vi "Keithley 6221-2182.vi"() -> ()   [LabVIEW 2018]
doc: "Stores specified measurements in buffer and reads the contents of the buffer as well as its statistics."
uses:
  <instrlib>/Keithley 622x LV 2009/Configure/Source/Typedefs/KE622x -- Current Range.ctl
  <instrlib>/Keithley 622x LV 2009/Configure/Source/Typedefs/KE622x -- Current Ranges.ctl
  <instrlib>/Keithley 622x LV 2009/Configure/Source/Typedefs/KE622x -- Lin Log Sweep Params.ctl
  <instrlib>/Keithley 622x LV 2009/Configure/Source/Typedefs/KE622x -- Source Delay.ctl
  <instrlib>/Keithley 622x LV 2009/Configure/Source/Typedefs/KE622x -- Current Level.ctl
  <instrlib>/Keithley 622x LV 2009/Typedefs/KE622x -- On Off Control.ctl
  <instrlib>/Keithley 622x LV 2009/Configure/Source/Typedefs/KE622x -- Voltage Limit.ctl
  <instrlib>/Keithley 622x LV 2009/Configure/Output/Typedefs/KE6221 -- Output Response.ctl
  <instrlib>/Keithley 622x LV 2009/Configure/Source/Typedefs/KE622x -- Sweep Type.ctl
  <instrlib>/Keithley 622x LV 2009/Configure/Trigger/Typedefs/KE6221 -- Arm Trig Wave Trig Params.ctl
  <instrlib>/Keithley 622x LV 2009/Configure/Trigger/Low Level/Typedefs/KE622x -- Arm Source.ctl
  <instrlib>/Keithley 622x LV 2009/Configure/Trigger/Low Level/Typedefs/KE622x -- Trig Link Line.ctl
  <instrlib>/Keithley 622x LV 2009/Configure/Trigger/Low Level/Typedefs/KE622x -- Arm Timer Interval.ctl
  <instrlib>/Keithley 622x LV 2009/Configure/Trigger/Low Level/Typedefs/KE622x -- Arm Output Mode.ctl
  <instrlib>/Keithley 622x LV 2009/Configure/Trigger/Low Level/Typedefs/KE622x -- Trig Source.ctl
  <instrlib>/Keithley 622x LV 2009/Configure/Trigger/Low Level/Typedefs/KE622x -- Trig Output Mode.ctl
  <instrlib>/Keithley 622x LV 2009/Configure/6221 Wave/Low Level/Typedefs/KE6221 -- Wave Extern Trig Link In Line.ctl
  <instrlib>/Keithley 622x LV 2009/Configure/6221 Wave/Low Level/Typedefs/KE6221 -- Wave Inactive Level.ctl
  <instrlib>/Keithley 622x LV 2009/Configure/6221 Wave/Low Level/Typedefs/KE6221 -- Wave Phase Marker.ctl
  <instrlib>/Keithley 622x LV 2009/Utility/Typedefs/KE622x -- Instrument Type.ctl
  <vilib>/Analysis/baseanly.llb/Mean (DBL).vi
  <instrlib>/Keithley 2182/Keithley 2182.lvlib
  <instrlib>/Keithley 622x LV 2009/Keithley 622x.lvlib
  <vilib>/Analysis/NI_AALBase.lvlib
panel:
  out "tdms file out":refnum<k34>
  in  "Tab Control":enum32{"Sweep", "Manual"}(tab)
  out "Volt":dbl[](array[numeric])=[0.00822021982, 0.00821965962, 0.0082210601, 0.00822078001, 0.00822218049, 0.00740205868, 0.00740121839, 0.00740093829, 0.00740121839, 0.00740149848, 0.00658025701, 0.00658025701, 0.00657969682, 0.00657969682, 0.0065805371, 0.00575845594, 0.00575873604, 0.00575845594, 0.00575817585, 0.00575845594, 0.00493441388, 0.00493441388, 0.00493413379, 0.00493413379, 0.00493385369, 0.00410897185, 0.00410869176, 0.00410925195, 0.00410897185, 0.00410925195, 0.00328605065, 0.00328605065, 0.00328577055, 0.00328605065, 0.00328605065, 0.00246284907, 0.00246284907, 0.00246228888, 0.00246228888, 0.00246312917, 0.00163992774, 0.00163992774, 0.00163964764, 0.00164048793, 0.00163992779, 0.000819247112, 0.000819527208, 0.000819247112, 0.0008200874, 0.0008200874, -3.1313761e-07, -3.1313761e-07, -1.15341924e-06, 2.47050147e-07, -5.93231488e-07, -0.000819307622, -0.000820708091, -0.000820708091, -0.000819867809, -0.000820427997, -0.00164222329, -0.00164222329, -0.00164222329, -0.00164222329, -0.0016419432, -0.00246345839, -0.00246429867, -0.00246429867, -0.00246429867, -0.00246485885, -0.00328581407, -0.00328637426, -0.00328693445, -0.00328749463, -0.00328721454, -0.00410620902, -0.00410620902, -0.0041067692, -0.00410760949, -0.0041070493, -0.00492884488, -0.00492912497, -0.00492884488, -0.00492884488, -0.00492912497, -0.00575232068, -0.00575232068, -0.0057517605, -0.0057514804, -0.0057514804, -0.00657355556, -0.00657355556, -0.00657299537, -0.00657355556, -0.00657383565, -0.00739815111, -0.00739787102, -0.00739843121, -0.00739843121, -0.00739843121, -0.00822358801, -0.00822358801, -0.00822470839, -0.0082238681, -0.00822442829]
  in  "Measurement (0: Voltage Channel 1)":i32(ring) items=["Voltage Channel 1", "Voltage Channel 2", "Temperature Channel 1", "Temperature Channel 2"]
  out "XY Graph":cluster{"Y":dbl[], "Y":dbl[]}[](graph)=[{"Y"=[-0.1, -0.1, -0.1, -0.1, -0.1, -0.09000000000000001, -0.09000000000000001, -0.09000000000000001, -0.09000000000000001, -0.09000000000000001, -0.08, -0.08, -0.08, -0.08, -0.08, -0.07, -0.07, -0.07, -0.07, -0.07, -0.060000000000000005, -0.060000000000000005, -0.060000000000000005, -0.060000000000000005, -0.060000000000000005, -0.05, -0.05, -0.05, -0.05, -0.05, -0.04000000000000001, -0.04000000000000001, -0.04000000000000001, -0.04000000000000001, -0.04000000000000001, -0.03, -0.03, -0.03, -0.03, -0.03, -0.020000000000000004, -0.020000000000000004, -0.020000000000000004, -0.020000000000000004, -0.020000000000000004, -0.010000000000000009, -0.010000000000000009, -0.010000000000000009, -0.010000000000000009, -0.010000000000000009, 0.0, 0.0, 0.0, 0.0, 0.0, 0.009999999999999995, 0.009999999999999995, 0.009999999999999995, 0.009999999999999995, 0.009999999999999995, 0.01999999999999999, 0.01999999999999999, 0.01999999999999999, 0.01999999999999999, 0.01999999999999999, 0.03, 0.03, 0.03, 0.03, 0.03, 0.04000000000000001, 0.04000000000000001, 0.04000000000000001, 0.04000000000000001, 0.04000000000000001, 0.04999999999999999, 0.04999999999999999, 0.04999999999999999, 0.04999999999999999, 0.04999999999999999, 0.06, 0.06, 0.06, 0.06, 0.06, 0.07, 0.07, 0.07, 0.07, 0.07, 0.07999999999999999, 0.07999999999999999, 0.07999999999999999, 0.07999999999999999, 0.07999999999999999, 0.09, 0.09, 0.09, 0.09, 0.09, 0.1, 0.1, 0.1, 0.1, 0.1], "Y"=[0.00822021982, 0.00821965962, 0.0082210601, 0.00822078001, 0.00822218049, 0.00740205868, 0.00740121839, 0.00740093829, 0.00740121839, 0.00740149848, 0.00658025701, 0.00658025701, 0.00657969682, 0.00657969682, 0.0065805371, 0.00575845594, 0.00575873604, 0.00575845594, 0.00575817585, 0.00575845594, 0.00493441388, 0.00493441388, 0.00493413379, 0.00493413379, 0.00493385369, 0.00410897185, 0.00410869176, 0.00410925195, 0.00410897185, 0.00410925195, 0.00328605065, 0.00328605065, 0.00328577055, 0.00328605065, 0.00328605065, 0.00246284907, 0.00246284907, 0.00246228888, 0.00246228888, 0.00246312917, 0.00163992774, 0.00163992774, 0.00163964764, 0.00164048793, 0.00163992779, 0.000819247112, 0.000819527208, 0.000819247112, 0.0008200874, 0.0008200874, -3.1313761e-07, -3.1313761e-07, -1.15341924e-06, 2.47050147e-07, -5.93231488e-07, -0.000819307622, -0.000820708091, -0.000820708091, -0.000819867809, -0.000820427997, -0.00164222329, -0.00164222329, -0.00164222329, -0.00164222329, -0.0016419432, -0.00246345839, -0.00246429867, -0.00246429867, -0.00246429867, -0.00246485885, -0.00328581407, -0.00328637426, -0.00328693445, -0.00328749463, -0.00328721454, -0.00410620902, -0.00410620902, -0.0041067692, -0.00410760949, -0.0041070493, -0.00492884488, -0.00492912497, -0.00492884488, -0.00492884488, -0.00492912497, -0.00575232068, -0.00575232068, -0.0057517605, -0.0057514804, -0.0057514804, -0.00657355556, -0.00657355556, -0.00657299537, -0.00657355556, -0.00657383565, -0.00739815111, -0.00739787102, -0.00739843121, -0.00739843121, -0.00739843121, -0.00822358801, -0.00822358801, -0.00822470839, -0.0082238681, -0.00822442829]}]
  in  "Autorange (T: Enable)":bool=TRUE
  in  "Range Value (10)":dbl=10.0
  in  "Voltage Resolution (8)":i32=8
  in  "Current Range In":T1={"Auto Range?"=FALSE, "Man / Selected\nRange"=enum."100mA"}
  in  "Lin Log Sweep Params In":T3={"Sweep Type"=enum."Linear", "Source Delay (s)"=2.0, "Range Method"=enum."Fixed", "Num Sweeps"=enum."Sweep Count", "Sweep Count"=1, "Start Level (A)"=-0.1, "Stop Level (A)"=0.1, "Step Level (A)"=0.01, "Num Steps"=21, "Abort On\nCompliance?"=FALSE} {"Num Steps" min=1 max=65535; "Step Level (A)" min=-0.105 max=0.105 format="%.4p"; "Stop Level (A)" min=-0.105 max=0.105 format="%.4p"; "Start Level (A)" min=-0.105 max=0.105 format="%.4p"; "Sweep Count" min=1 max=9999; "Source Delay (s)" min=0.001 max=1000.0 step=0.001 format="%.3f"}
  in  "# Meas per step":i32=5
  out "Metadata":T6={"Units"="VDC", "Channel"=1, "Channel Type"="INTERNAL"}
  out "length 2":i32=105
  out "Current":dbl[](array[numeric])=[0.00823056931, 0.0082311295, 0.0082314096, 0.00823168969, 0.0082311295, -3.3038258e-08, -3.1313168e-07, -3.1313168e-07, -5.93225102e-07, -1.15341195e-06, -0.00822665531, -0.00822609513, -0.00822609513, -0.00822665531, -0.00822609513]
  out "length":i32=105
  in  "Output State":T7=enum."On"
  in  "Turn Off Output If Voltage Limit?":bool=TRUE
  out "Voltage Limit?":bool
  out "Interlock Tripped?":bool
  in  "Voltage Limit (V)":T8=5.0 min=0.1 max=105.0 step=0.01 format="%.2p"
  in  "Current Level (A)":T5=0.02 min=-0.105 max=0.105 format="%.4p"
  in  "Output Response":T9=enum."Slow"
  in  "Analog Filter State":T7
  in  "Current Range In 2":T1={"Auto Range?"=TRUE, "Man / Selected\nRange"=enum."2nA"}
  in  "stop":bool
  out "Output on?":bool=TRUE
  in  "Initiate Type (0: Immediate)":i32(ring) items=["Immediate", "Continuous"]
  out "Measurements":dbl[](array[numeric])=[-0.00164131953, -0.00164132201, -0.0016413518, -0.00164135614, -0.00164135366, -0.00164140207, -0.00164139897, -0.00164140889, -0.00164142069, -0.0016414597]
  in  "Buffer Size (10)":i32=10
  in  "Buffer Source (0: None)":i32(ring)=1 items=["None", "Measurements", "Math Calculation"]
  in  "Measurement (0: Voltage Channel 1) 2":i32(ring) items=["Voltage Channel 1", "Voltage Channel 2", "Temperature Channel 1", "Temperature Channel 2"]
  in  "Integration Rate (5)":dbl=1.0
  in  "Integration Rate Units (0: Line Cycles)":i32(ring) items=["Line Cycles", "Seconds"]
  in  "Selected Calculation Settings":enum32{"Linear Settings", "Percent Settings"}(tab)
  in  "Offset Value (0)":dbl
  in  "Scale Factor (1)":dbl=1.0
  in  "Units (MX)":string="MX"
  in  "Use Input Signal as Target Value (F: Disable)":bool
  in  "Target Value (1)":dbl=1.0
  in  "Math Calculation (0: Linear)":i32(ring) items=["Linear", "Percent"]
  in  "Selected Measurement Settings":enum32{"Voltage Settings", "Temp Settings"}(tab)=enum."Temp Settings"
  in  "Voltage Resolution (8) 2":i32=8
  in  "Range Value (10) 2":dbl=10.0
  in  "Autorange (T: Enable) 2":bool=TRUE
  in  "Sensor (1: Internal)":i32(ring)=1 items=["Thermocouple", "Internal"]
  in  "Reference Junction Type (0: Internal)":i32(ring) items=["Internal", "Simulated"]
  in  "Simulated Reference Temp (23 C)":dbl=23.0
  in  "Thermocouple Type (0: J)":i32(ring) items=["J", "K", "T", "E", "R", "S", "B", "N"]
  in  "Temperature Resolution (6)":i32=6
  in  "Unit (0: Celsius)":i32(ring) items=["Celsius", "Fahrenheit", "Kelvin"]
  out "XY Graph 2":cluster{"X":dbl[], "Y":dbl[]}[](graph)=[{"X"=[3634154561.485772, 3634154562.303772, 3634154563.182772, 3634154564.037772, 3634154564.896772, 3634154565.763772, 3634154566.636772, 3634154567.479772, 3634154568.339772, 3634154569.237772, 3634154570.094772, 3634154570.939772, 3634154571.892772, 3634154572.709772, 3634154573.511772, 3634154574.369772, 3634154575.274772, 3634154576.125772, 3634154576.960772, 3634154577.801772, 3634154578.658772, 3634154579.492772, 3634154580.341772, 3634154581.174772, 3634154582.025772, 3634154582.857772, 3634154583.706772, 3634154584.541772, 3634154585.376772, 3634154586.181772, 3634154587.005772, 3634154587.869772, 3634154588.716772, 3634154589.555772, 3634154590.398772, 3634154591.315772, 3634154592.163772, 3634154593.027772, 3634154593.905772, 3634154594.757772, 3634154595.614772, 3634154596.470772, 3634154597.297772, 3634154598.146772, 3634154599.008772, 3634154599.897772, 3634154600.766772, 3634154601.606772, 3634154602.448772, 3634154603.295772, 3634154604.164772, 3634154605.032772, 3634154605.863772, 3634154606.695772, 3634154607.553772, 3634154608.406772, 3634154609.261772, 3634154610.115772, 3634154610.999772, 3634154611.898772, 3634154612.758772, 3634154613.654772, 3634154614.486772, 3634154615.311772, 3634154616.161772, 3634154616.997772, 3634154617.853772, 3634154618.701772, 3634154619.537772, 3634154620.370772, 3634154621.236772, 3634154622.071772, 3634154622.897772, 3634154623.744772, 3634154624.594772, 3634154625.431772, 3634154626.289772, 3634154627.165772, 3634154628.039772, 3634154628.896772], "Y"=[6.714419513e-08, 7.117796388999999e-08, 6.925411786999999e-08, 7.179855940000001e-08, 7.570795384000001e-08, 6.689550554000002e-08, 6.615033896999999e-08, 7.248040024e-08, 6.66467944e-08, 7.248019181000001e-08, 7.167341972000001e-08, -0.0008212093023366601, -0.001642361878, -0.001642302666, -0.0016425070280000002, -0.0016426372790000001, -0.0016418216670000003, -0.0016411064359999998, -0.0016408055500000001, -0.00164062229, -0.0016405603680000002, -0.001640255471, -0.0016401012559999998, -0.001640932988, -0.001641709718, -0.0016417949600000003, -0.001641990694, -0.0016425602700000004, -0.001642962542, -0.001643020379, -0.001643063698, -0.0016432126540000002, -0.001642921969, -0.0016427625710000002, -0.0016425643539999999, -0.001642402515, -0.001642034878, -0.001641597088, -0.001641742526, -0.0016422704, -0.001641864116, -0.0016413054589999997, -0.001640804558, -0.0016398811829999999, -0.0016389855380000002, -0.0016388971519999997, -0.0016394337789999997, -0.001639557069, -0.0016398090269999998, -0.0016403630069999997, -0.0016410822090000003, -0.0016414387039999998, -0.0016414943759999999, -0.001641617997, -0.001641962501, -0.00164235192, -0.0016424170420000002, -0.001642482638, -0.001641888906, -0.001640921356, -0.0016406053350000002, -0.001640670214, -0.001640900889, -0.0016410445540000003, -0.00164120262, -0.001641145974, -0.001640773621, -0.00164026815, -0.0016400809620000002, -0.001639955479, -0.001640031716, -0.0016403619309999999, -0.001640644547, -0.001640697017, -0.001640906774, -0.0016411437610000003, -0.001641041116, -0.0016409511410000002, -0.0016411044320000002, -0.0016413793460000002]}]
  out "Measurement Metadata":T6={"Units"="VDC", "Channel"=1, "Channel Type"="INTERNAL"}
  in  "6221 VISA":refnum<visa-resource-name>="TCPIP0::192.168.1.2::1394::SOCKET"
  in  "2182a VISA":refnum<visa-resource-name>="COM16"
  # "Modes:\nSweep uses preset step parameters to \ntrigger measurements of current and \nvoltage\n\nManual allows for continuous voltage \nmeasurements and records each time\nthe current and output state are\nchanged\nThe changing states act as events to \ninfercurrent levels for specific voltage.\n\n**DO NOT SWITCH TABS WHILE RUNNING\n\n**SET SWEEP PARAMETERS\nBEFORE STARTING VI"
  # "Measurement Settings"
  # "Data"
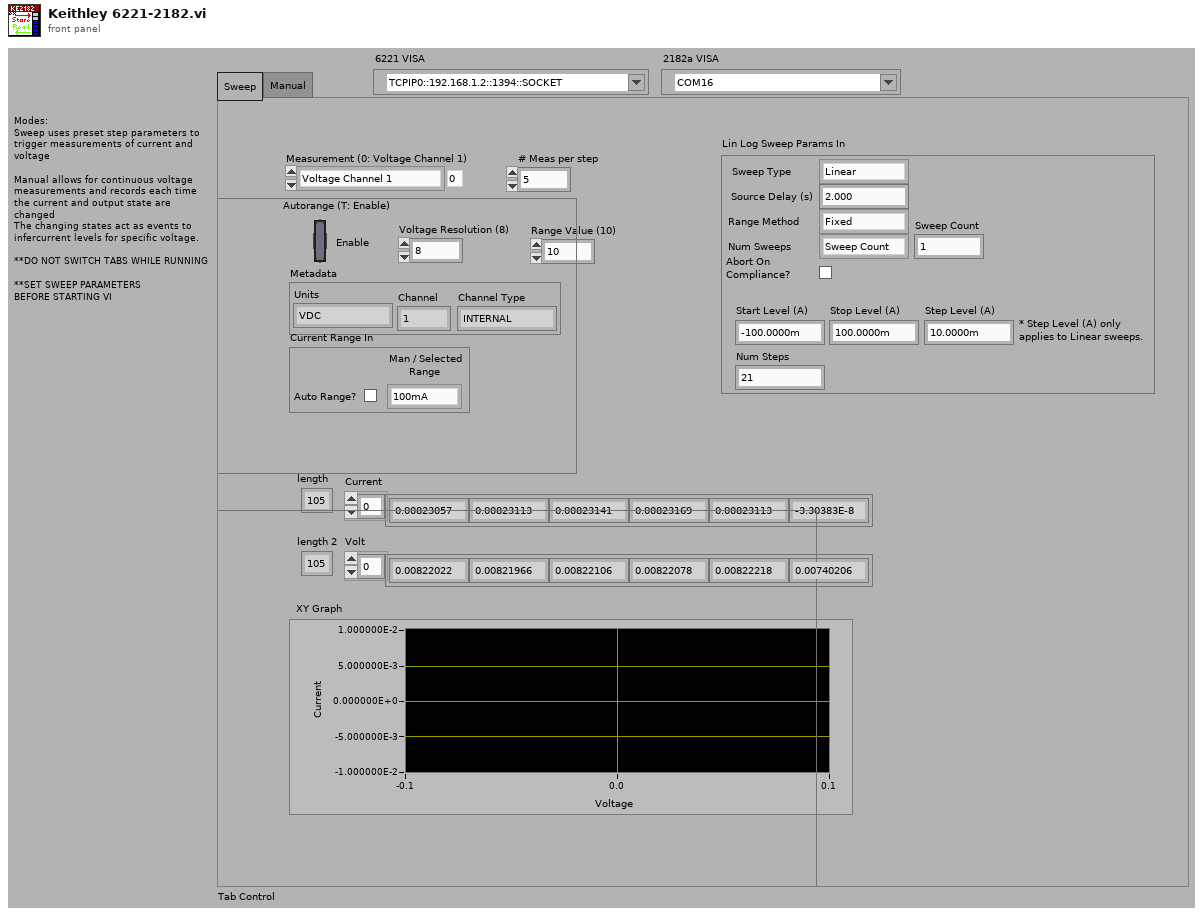
[diagram p1: front panel]
types:
  T1 = typedef "Keithley 622x.lvlib/KE622x -- Current Range.ctl" = cluster{"Auto Range?":bool, "Man / Selected\nRange":T2}
  T2 = typedef "Keithley 622x.lvlib/KE622x -- Current Ranges.ctl" = enum16{"2nA", "20nA", "200nA", "2uA", "20uA", "200uA", "2mA", "20mA", "100mA"}
  T3 = typedef "Keithley 622x.lvlib/KE622x -- Lin Log Sweep Params.ctl" = cluster{"Sweep Type":enum16{"Linear", "Log", "List"}, "Source Delay (s)":T4, "Range Method":enum16{"Auto", "Best", "Fixed"}, "Num Sweeps":enum16{"Sweep Count", "Infinite"}, "Sweep Count":u32, "Start Level (A)":T5, "Stop Level (A)":T5, "Step Level (A)":T5, "Num Steps":u32, "Abort On\nCompliance?":bool}
  T4 = typedef "Keithley 622x.lvlib/KE622x -- Source Delay.ctl" = dbl
  T5 = typedef "Keithley 622x.lvlib/KE622x -- Current Level.ctl" = dbl
  T6 = cluster{"Units":string, "Channel":i32, "Channel Type":string}
  T7 = typedef "Keithley 622x.lvlib/KE622x -- On Off Control.ctl" = enum16{"Off", "On"}
  T8 = typedef "Keithley 622x.lvlib/KE622x -- Voltage Limit.ctl" = dbl
  T9 = typedef "Keithley 622x.lvlib/KE6221 -- Output Response.ctl" = enum16{"Fast", "Slow"}
  T10 = typedef "Keithley 622x.lvlib/KE622x -- Instrument Type.ctl" = enum16{"KE6220", "KE6221"}
  T11 = typedef "Keithley 622x.lvlib/KE6221 -- Arm Trig Wave Trig Params.ctl" = cluster{"Arm Layer Input Trig Bypassed?":bool, "Arm Layer Input Trig Source":T12, "Arm Layer Input Trig Link Line":T13, "Arm Layer Input Trig Timer Interval (s)":T14, "Arm Layer Output Trig Mode":T15, "Arm Layer Output Trig Link Line":T13, "Trig Layer Input Trig Source":T16, "Trig Layer Input Trig Link Line":T13, "Trig Layer Output Trig Mode":T17, "Trig Layer Output Trig Link Line":T13, "6221 Wave Input Trig Enabled?":bool, "6221 Wave Input Trig Link Line":T18, "6221 Wave Inactive Level (%)":T19, "6221 Wave Ingore Input Retrigs?":bool, "6221 Phase Marker Output Trig Enabled?":bool, "6221 Phase Marker (deg)":T20, "6221 Phase Marker Output Trig Link Line":T13}
  T12 = typedef "Keithley 622x.lvlib/KE622x -- Arm Source.ctl" = enum16{"Immediate", "Bus (*TRG)", "Timer", "Manual", "Trigger Link", "SOT Falling Edge", "SOT Rising Edge", "SOT Either Edge"}
  T13 = typedef "Keithley 622x.lvlib/KE622x -- Trig Link Line.ctl" = enum16{"1", "2", "3", "4", "5", "6"}
  T14 = typedef "Keithley 622x.lvlib/KE622x -- Arm Timer Interval.ctl" = dbl
  T15 = typedef "Keithley 622x.lvlib/KE622x -- Arm Output Mode.ctl" = enum16{"No Trig Out", "Trig Out On Enter Arm", "Trig Out On Exit Arm"}
  T16 = typedef "Keithley 622x.lvlib/KE622x -- Trig Source.ctl" = enum16{"Immediate", "Trigger Link"}
  T17 = typedef "Keithley 622x.lvlib/KE622x -- Trig Output Mode.ctl" = enum16{"No Trig Out", "Source Turn On", "After Source Delay"}
  T18 = typedef "Keithley 622x.lvlib/KE6221 -- Wave Extern Trig Link In Line.ctl" = enum16{"None", "1", "2", "3", "4", "5", "6"}
  T19 = typedef "Keithley 622x.lvlib/KE6221 -- Wave Inactive Level.ctl" = dbl
  T20 = typedef "Keithley 622x.lvlib/KE6221 -- Wave Phase Marker.ctl" = dbl
  T21 = enum16{"open", "open or create", "create or replace", "create", "open (read-only)"}
  T22 = typedef "Keithley 622x.lvlib/KE622x -- Sweep Type.ctl" = enum16{"Linear", "Log", "List"}
  T23 = cluster{"Units":string, "Channel":i32, "Channel Type":string}[]
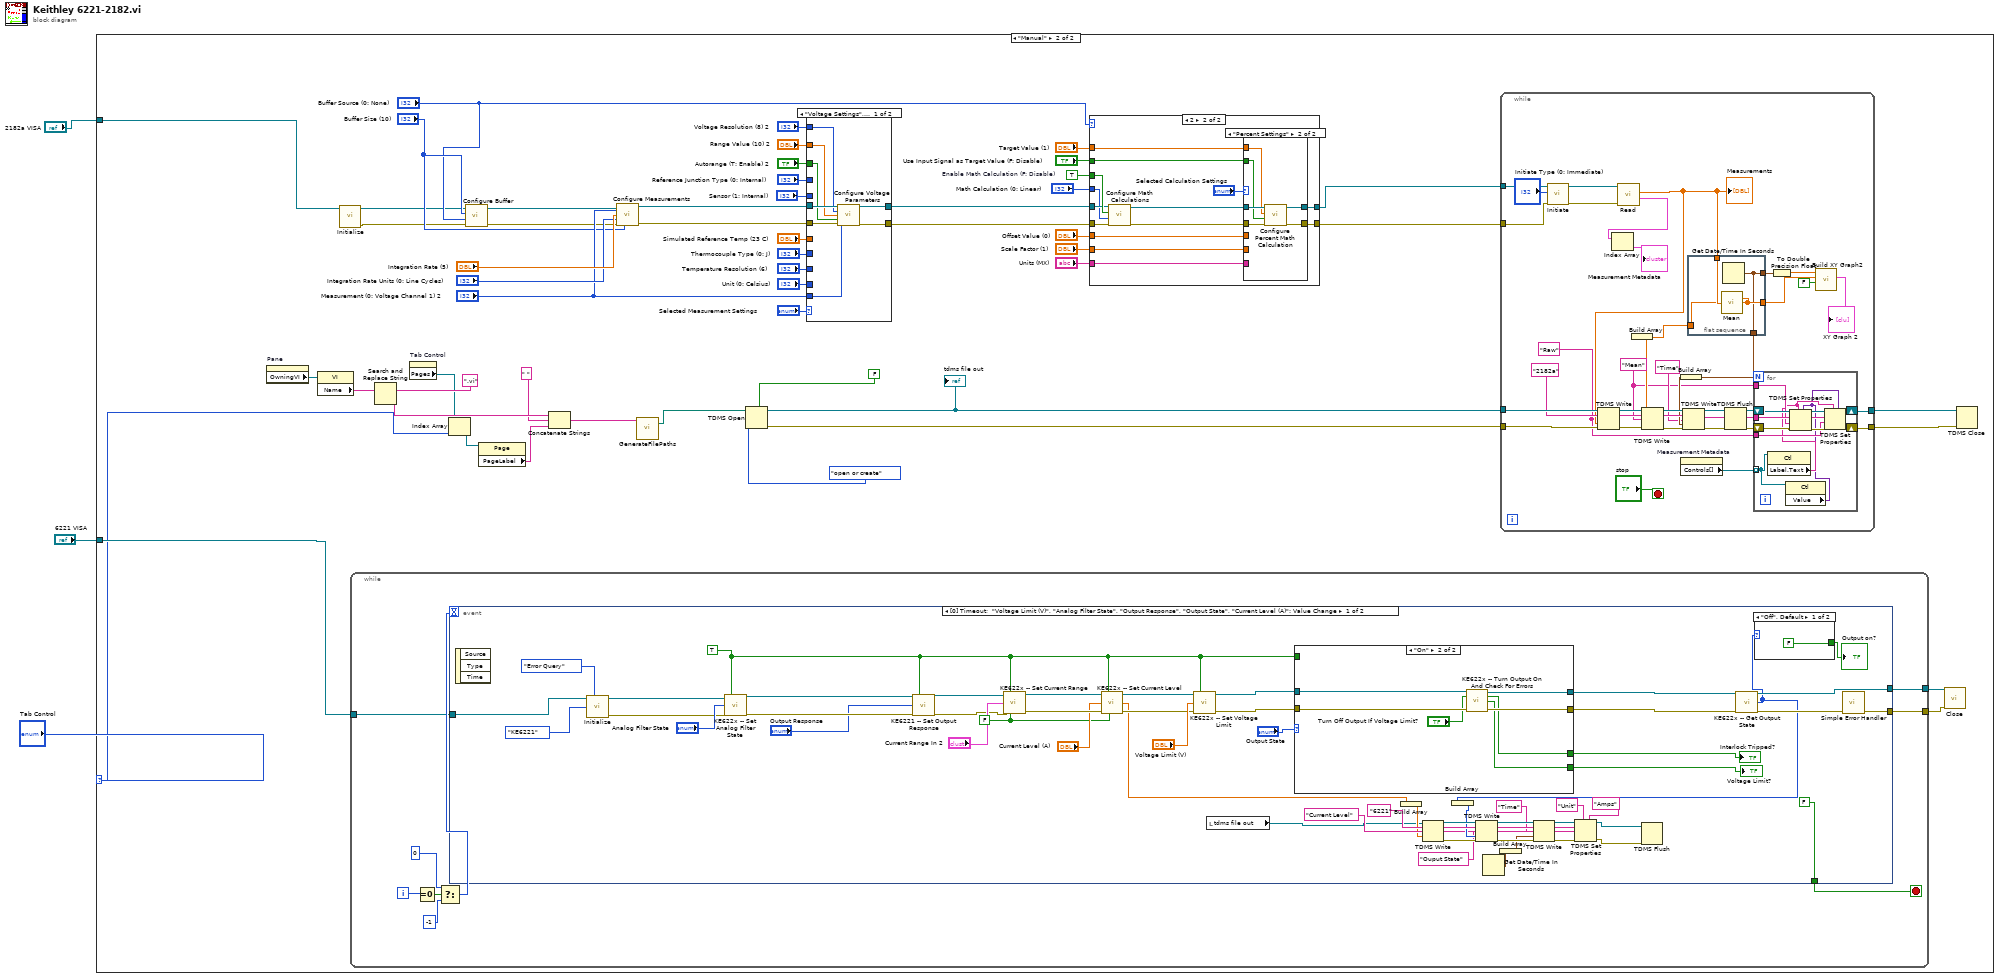
[diagram p0: block diagram]
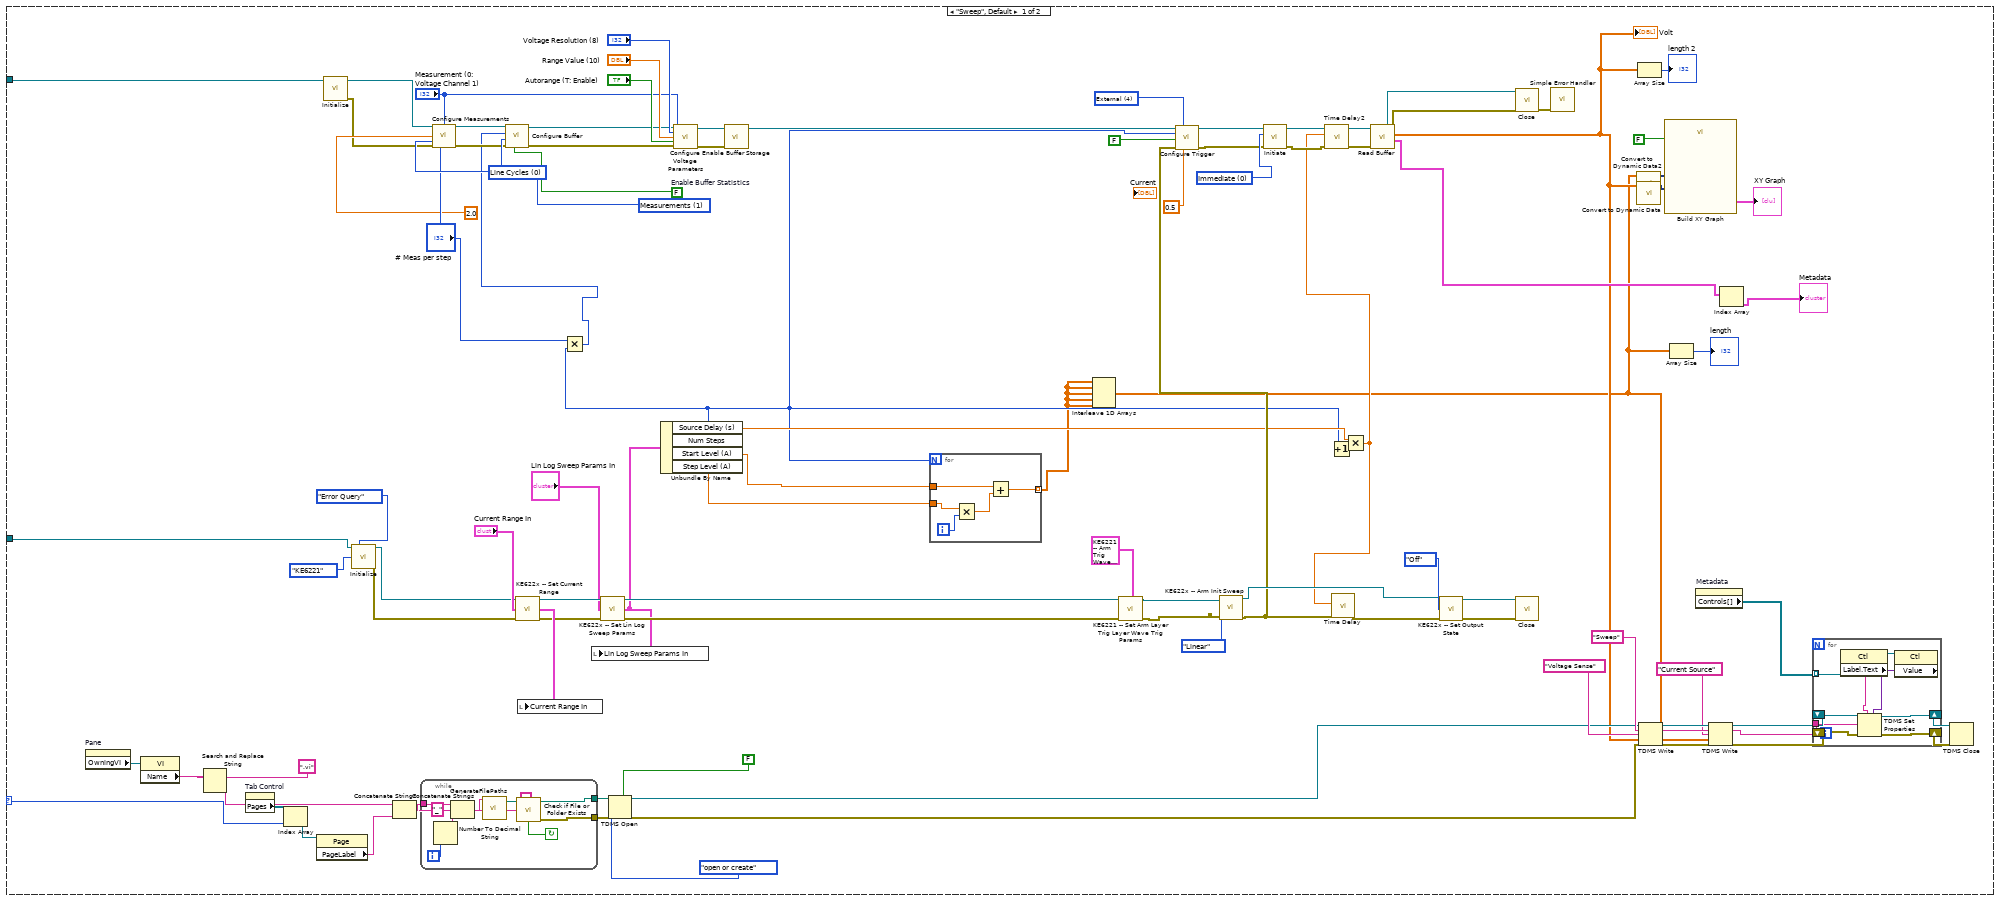
[diagram p2: hidden frame]
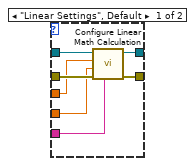
[diagram p4: hidden frame]
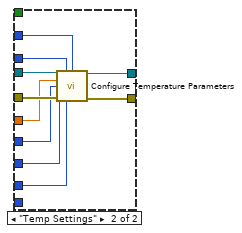
[diagram p5: hidden frame]
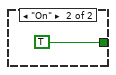
[diagram p6: hidden frame]
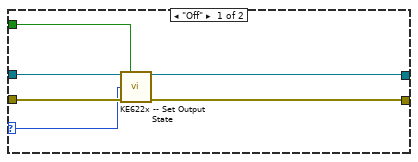
[diagram p7: hidden frame]
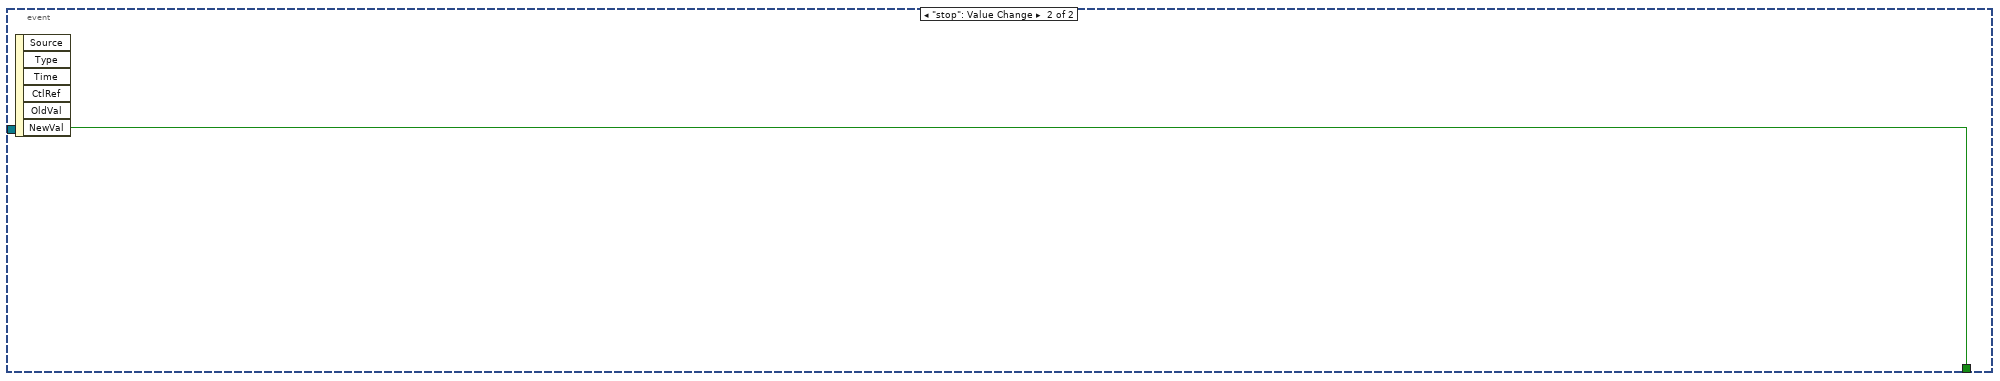
[diagram p8: hidden frame]
diagram:
  n1 = case shown="\"Manual\"" "Tab Control" {
    selector: "Tab Control" -> [w14 w135]
    tunnel: "6221 VISA" -> [w11 w178]
    tunnel: "2182a VISA" -> [w10 w179]
    frame "Sweep", Default {
      w99 = 1 items=["None", "Measurements", "Math Calculation"] ("Buffer Source (0: None)")
      w103 = 0 items=["Line Cycles", "Seconds"] ("Integration Rate Units (0: Line Cycles)")
      w84 = 0 items=["Immediate", "Continuous"] ("Initiate Type (0: Immediate)")
      w89 = 4 items=["Immediate", "Timer", "Manual", "Bus", "External"] ("Trigger Source (0: Immediate)")
      w97 = FALSE  # Enable Buffer Statistics
      n2 = property on="Pane" class="Pane"() -> ("OwningVI"=w25:refnum<vi>)  [unwired: 2 in, 2 out]
      n3 = property class="VI"(reference=w25) -> ("Name"=w23:string)  [unwired: 1 in, 2 out]
      n4 = Search and Replace String(input string=w23, search string=".vi") -> (result string=w26:string)  [unwired: 6 in, 3 out]
      n5 = property on="Tab Control" class="TabCtl (strict)"() -> ("Pages"=w16:refnum<vi>[])  [unwired: 2 in, 2 out]
      n6 = Index Array(array=w16, index=w14) -> (element=w15:refnum<vi>)
      n7 = property on="Property Node" class="Page"(reference=w15) -> ("PageLabel"=w13:string)  [unwired: 1 in, 2 out]
      n8 = call <instrlib>:"Initialize.vi"("VISA resource name"=w10) -> ("error out"=w18:errorcluster, "VISA resource name out"=w17:refnum<visa-resource-name>)  [unwired: 9 in]
      n9 = call <instrlib>:"Initialize.vi"("VISA resource name"=w11, "Error Queue Option"=enum16{"Clear Error Queue", "Error Query"}."Error Query", "Instrument Type"=KE622x_--_Instrument_Type."KE6221") -> ("VISA resource name out"=w20:refnum<visa-resource-name>, "error out"=w19:errorcluster)  [unwired: 11 in]
      n10 = Concatenate Strings(w26, " " ("string"), w13) -> (w22:string)
      n11 = while {
        tunnel: [w111] -> w28
        tunnel: [w110] -> w27
        tunnel: w22 -> [w108]
        i -> [w105]
        stop <- w112 continue-if-true
        n12 = Number To Decimal String(number=w105) -> (decimal integer string=w104:string)  [unwired: 1 in]
        n13 = Concatenate Strings(w108, "_" ("string"), w104) -> (w107:string)
        n14 = call "GenerateFilePaths.vi"("Device Name"=w107) -> ("Path"=w109:path)  [unwired: 4 in]
        n15 = call <vilib>:"Check if File or Folder Exists.vi"("path"=w109) -> ("error out"=w111:errorcluster, "file or folder exists?"=w112:bool, "dup path"=w110:path)  [unwired: 8 in]
      }
      n16 = call <instrlib>:"Configure Measurements.vi"("VISA resource name"=w17, "Measurement (0: Voltage Channel 1)"="Measurement (0: Voltage Channel 1)", "Integration Rate (5)"=2.0, "Integration Rate Units (0: Line Cycles)"=w103, "error in (no error)"=w18, "Sample Count (1)"="# Meas per step") -> ("VISA resource name out"=w57:refnum<visa-resource-name>, "error out"=w56:errorcluster)  [unwired: 8 in]
      n17 = call <instrlib>:"KE622x -- Set Current Range.vi"("Resource In"=w20, "Current Range In"="Current Range In", "error in (no error)"=w19) -> ("Resource Out (dupl)"=w88:refnum<visa-resource-name>, "Current Range Out"=w94:T1, "error out"=w87:errorcluster)  [unwired: 10 in]
      n18 = local write "Current Range In"(w94) -> ()
      n19 = call <instrlib>:"KE622x -- Set Lin Log Sweep Params.vi"("Resource In"=w88, "Lin Log Sweep Params In"="Lin Log Sweep Params In", "error in (no error)"=w87) -> ("Resource Out (dupl)"=w68:refnum<visa-resource-name>, "Lin Log Sweep Params Out"=w59:T3, "error out"=w69:errorcluster)  [unwired: 10 in]
      n20 = local write "Lin Log Sweep Params In"(w59) -> ()
      n21 = TDMS Open(5:FALSE ("create index file? (T)"), 8:w28, 10:T21."open or create" ("operation (0:open)"), 11:w27) -> (0:w37:errorcluster, 3:w38:refnum<k34>)  [unwired: 3 in]
      n22 = Unbundle By Name(w59) -> ("Source Delay (s)"=w61:T4, "Num Steps"=w50:u32, "Start Level (A)"=w49:T5, "Step Level (A)"=w48:T5)
      n23 = Multiply(x="# Meas per step", y=w50) -> (x*y=w52:u32)
      n24 = call <instrlib>:"Configure Buffer.vi"("Enable Buffer Statistics (0: Disable)"=w97, "error in (no error)"=w56, "Buffer Source (0: None)"=w99, "Buffer Size (2)"=w52, "VISA resource name"=w57) -> ("error out"=w55:errorcluster, "VISA resource name out"=w54:refnum<visa-resource-name>)  [unwired: 5 in]
      n25 = call <instrlib>:"Configure Voltage Parameters.vi"("VISA resource name"=w54, "Measurement (1: Voltage Channel 1)"="Measurement (0: Voltage Channel 1)", "Voltage Resolution (8)"="Voltage Resolution (8)", "Range Value (12)"="Range Value (10)", "Autorange (T: Enable)"="Autorange (T: Enable)", "error in (no error)"=w55) -> ("VISA resource name out"=w63:refnum<visa-resource-name>, "error out"=w62:errorcluster)  [unwired: 8 in]
      n26 = call <instrlib>:"Enable Buffer Storage.vi"("error in (no error)"=w62, "VISA resource name"=w63) -> ("VISA resource name out"=w64:refnum<visa-resource-name>)  [unwired: 8 in, 1 out]
      n27 = for {
        N: w50 -> [_]
        tunnel: w49 -> [w124]
        tunnel: w48 -> [w125]
        tunnel: [w122] -> w47 mode=indexing
        i -> [w126]
        n28 = Multiply(x=w125, y=w126) -> (x*y=w123:T5)
        n29 = Add(x=w124, y=w123) -> (x+y=w122:T5)
      }
      n30 = Interleave 1D Arrays(w47, w47, w47, w47, w47) -> (w4:T5[])
      n31 = call <instrlib>:"KE6221 -- Set Arm Layer Trig Layer Wave Trig Params.vi"("Resource In"=w68, "6221 Arm Trig Wave Trig Params In"=T11 {"Arm Layer Input Trig Bypassed?"=FALSE, "Arm Layer Input Trig Source"=enum."Timer", "Arm Layer Input Trig Link Line"=enum."1", "Arm Layer Input Trig Timer Interval (s)"=2.0, "Arm Layer Output Trig Mode"=enum."Trig Out On Enter Arm", "Arm Layer Output Trig Link Line"=enum."2", "Trig Layer Input Trig Source"=enum."Trigger Link", "Trig Layer Input Trig Link Line"=enum."1", "Trig Layer Output Trig Mode"=enum."Source Turn On", "Trig Layer Output Trig Link Line"=enum."2", "6221 Wave Input Trig Enabled?"=FALSE, "6221 Wave Input Trig Link Line"=enum."None", "6221 Wave Inactive Level (%)"=0.0, "6221 Wave Ingore Input Retrigs?"=FALSE, "6221 Phase Marker Output Trig Enabled?"=FALSE, "6221 Phase Marker (deg)"=180.0, "6221 Phase Marker Output Trig Link Line"=enum."6"}, "error in (no error)"=w69) -> ("Resource Out (dupl)"=w67:refnum<visa-resource-name>, "error out"=w66:errorcluster)  [unwired: 10 in, 1 out]
      n32 = call <instrlib>:"KE622x -- Arm Init Sweep.vi"("Resource In"=w67, "Sweep Type"=KE622x_--_Sweep_Type."Linear", "error in (no error)"=w66) -> ("Resource Out (dupl)"=w86:refnum<visa-resource-name>, "error out"=w71:errorcluster)  [unwired: 11 in]
      n33 = call <instrlib>:"Configure Trigger.vi"("VISA resource name"=w64, "Trigger Source (0: Immediate)"=w89, "Trigger Count (1)"=w50, "Autodelay (T: Enable)"=FALSE, "error in (no error)"=w71, "Trigger Delay (0 s)"=0.5) -> ("VISA resource name out"=w82:refnum<visa-resource-name>, "error out"=w83:errorcluster)  [unwired: 8 in]
      n34 = call <instrlib>:"Initiate.vi"("error in (no error)"=w83, "Initiate Type (0: Immediate)"=w84, "VISA resource name"=w82) -> ("error out"=w72:errorcluster, "VISA resource name out"=w80:refnum<visa-resource-name>)  [unwired: 7 in]
      n35 = Increment(x=w50) -> (x+1=w58:u32)
      n36 = Multiply(x=w61, y=w58) -> (x*y=w51:T4)
      n37 = call "Time Delay2"("error in (no error)"=w72, "Delay Time (s)"=w51) -> ("error out"=w74:errorcluster)  [unwired: 9 in]
      n38 = call "Time Delay"("error in (no error)"=w71, "Delay Time (s)"=w51) -> ("error out"=w90:errorcluster)  [unwired: 9 in]
      n39 = call <instrlib>:"Read Buffer.vi"("error in (no error)"=w74, "VISA resource name"=w80) -> ("error out"=w81:errorcluster, "Buffer Metadata"=w36:T23, "Buffer"=w9:dbl[], "VISA resource name out"=w79:refnum<visa-resource-name>)  [unwired: 6 in]
      "Volt" <- w9
      n40 = call <instrlib>:"KE622x -- Set Output State.vi"("Resource In"=w86, "Output State"=KE622x_--_On_Off_Control."Off", "error in (no error)"=w90) -> ("Resource Out (dupl)"=w92:refnum<visa-resource-name>, "error out"=w91:errorcluster)  [unwired: 11 in]
      n41 = call <instrlib>:"Close.vi"("error in (no error)"=w81, "VISA resource name"=w79) -> ("error out"=w96:errorcluster)  [unwired: 9 in]
      n42 = call <instrlib>:"Close.vi"("VISA resource name"=w92, "error in (no error)"=w91) -> ()  [unwired: 13 in, 1 out]
      n43 = call <vilib>:"Simple Error Handler.vi"("error in (no error)"=w96) -> ()  [unwired: 4 in, 5 out]
      n44 = call "Convert to Dynamic Data2"("Array"=w4) -> ("Dynamic Data Type"=w75:dynamicdata)  [unwired: 3 in]
      n45 = call "Convert to Dynamic Data"("Array"=w9) -> ("Dynamic Data Type"=w77:dynamicdata)  [unwired: 3 in]
      n46 = Array Size(array=w9) -> (size(s)=→"length 2":i32)
      n47 = TDMS Write(0:w38, 5:"Sweep" ("group name in (Untitled)"), 7:"Voltage Sense", 9:w9, 11:w37) -> (4:w44:refnum<k34>, 6:w43:string, 15:w42:errorcluster)  [unwired: 1 in, 1 out]
      n48 = call "Build XY Graph"("Reset"=FALSE, "Y Input"=w77, "X Input"=w75) -> ("XY Graph"=→"XY Graph":cluster{"X":dbl[], "Y":dbl[]}[])  [unwired: 7 in, 1 out]
      n49 = Array Size(array=w4) -> (size(s)=→"length":i32)
      n50 = property on="Metadata" class="Clust (strict)"() -> ("Controls[]"=w35:refnum<vi>[])  [unwired: 2 in, 2 out]
      n51 = TDMS Write(0:w44, 5:w43, 7:"Current Source", 9:w4, 11:w42) -> (4:w32:refnum<k34>, 6:w33:string, 15:w34:errorcluster)  [unwired: 1 in, 1 out]
      n52 = Index Array(array=w36) -> (element=→"Metadata":T6)  [unwired: 1 in]
      n53 = for {
        tunnel: w35 -> [w121] mode=indexing
        tunnel: w33 -> [w119]
        shift-right: [w117] -> w31
        shift-left: w32 -> [w118]
        shift-right: [w116] -> w30
        shift-left: w34 -> [w120]
        n54 = property class="Ctl"(reference=w121) -> (reference out=w113:refnum<vi>, "Label.Text"=w114:string)  [unwired: 1 in, 1 out]
        n55 = property class="Ctl"(reference=w113) -> ("Value"=w115:variant)  [unwired: 1 in, 2 out]
        n56 = TDMS Set Properties(5:w115, 7:w114, 8:w120, 10:w119, 11:w118) -> (0:w116:errorcluster, 3:w117:refnum<k34>)  [unwired: 1 in, 2 out]
      }
      n57 = TDMS Close(8:w30, 11:w31) -> ()  [unwired: 2 out]
    }
    frame "Manual" {
      w162 = TRUE  # Enable Math Calculation (F: Disable)
      n58 = property on="Pane" class="Pane"() -> ("OwningVI"=w142:refnum<vi>)  [unwired: 2 in, 2 out]
      n59 = property class="VI"(reference=w142) -> ("Name"=w140:string)  [unwired: 1 in, 2 out]
      n60 = call <instrlib>:"Initialize.vi"("VISA resource name"=w179) -> ("error out"=w146:errorcluster, "VISA resource name out"=w147:refnum<visa-resource-name>)  [unwired: 9 in]
      n61 = while {
        tunnel: w178 -> [w283]
        tunnel: [w282] -> w177
        tunnel: [w281] -> w176
        i -> [w288]
        stop <- w289 stop-if-true
        n62 = Equal To 0?(x=w288) -> (x = 0?=w287:bool)
        n63 = Select(t=0, s=w287, f=-1) -> (s? t:f=w284:i32)
        n64 = event shown="[0] Timeout;  \"Voltage Limit (V)\", \"Analog Filter State\", \"Output Response\", \"Output State\", \"Current Level (A)\": Value Change" {
          selector: _ -> [_ _]
          dyn-events: _ -> [_ _]
          timeout: w284 -> [_ _]
          tunnel: [FALSE w362] -> w289
          tunnel: w283 -> [w322 _]
          tunnel: [w320 _] -> w282
          tunnel: [w316 _] -> w281
          event Timeout; Value Change {
            w330 = TRUE ("Check For SCPI Errors? (T)")
            w337 = FALSE ("Read Back Set Values? (T)")
            n65 = event-data() -> ()  [unwired: 1 in, 3 out]
            n66 = call <instrlib>:"Initialize.vi"("VISA resource name"=w322, "Error Queue Option"=enum16{"Clear Error Queue", "Error Query"}."Error Query", "Instrument Type"=KE622x_--_Instrument_Type."KE6221") -> ("VISA resource name out"=w325:refnum<visa-resource-name>, "error out"=w324:errorcluster)  [unwired: 11 in]
            n67 = call <instrlib>:"KE622x -- Set Analog Filter State.vi"("Resource In"=w325, "Check For SCPI Errors? (T)"=w330, "Analog Filter State"="Analog Filter State", "error in (no error)"=w324) -> ("Resource Out (dupl)"=w344:refnum<visa-resource-name>, "error out"=w343:errorcluster)  [unwired: 10 in]
            n68 = call <instrlib>:"KE6221 -- Set Output Response.vi"("Resource In"=w344, "Check For SCPI Errors? (T)"=w330, "KE6221 Output Response"="Output Response", "error in (no error)"=w343) -> ("Resource Out (dupl)"=w341:refnum<visa-resource-name>, "error out"=w342:errorcluster)  [unwired: 10 in]
            n69 = call <instrlib>:"KE622x -- Set Current Range.vi"("Resource In"=w341, "Check For SCPI Errors? (T)"=w330, "Current Range In"="Current Range In 2", "error in (no error)"=w342, "Read Back Set Values? (T)"=w337) -> ("Resource Out (dupl)"=w340:refnum<visa-resource-name>, "error out"=w339:errorcluster)  [unwired: 8 in, 1 out]
            n70 = call <instrlib>:"KE622x -- Set Current Level.vi"("Resource In"=w340, "Check For SCPI Errors? (T)"=w330, "Current Level (A) In"="Current Level (A)", "error in (no error)"=w339, "Read Back Set Value? (T)"=w337) -> ("Resource Out (dupl)"=w335:refnum<visa-resource-name>, "Current Level (A) Out"=w312:T5, "error out"=w334:errorcluster)  [unwired: 8 in]
            n71 = call <instrlib>:"KE622x -- Set Voltage Limit.vi"("Resource In"=w335, "Check For SCPI Errors? (T)"=w330, "Voltage Limit (V)"="Voltage Limit (V)", "error in (no error)"=w334) -> ("Resource Out (dupl)"=w333:refnum<visa-resource-name>, "error out"=w332:errorcluster)  [unwired: 10 in]
            n72 = local read "tdms file out"() -> (w308:refnum<k34>)
            n73 = case shown="\"On\"" "Output State" {
              selector: "Output State" -> [w352 _]
              tunnel: w333 -> [w354 w361]
              tunnel: w332 -> [w353 w360]
              tunnel: [w350 w358] -> w318
              tunnel: w330 -> [w351 _]
              tunnel: [_ w357] -> w329
              tunnel: [_ w356] -> w328
              tunnel: [w349 w355] -> w319
              frame "Off" {
                n74 = call <instrlib>:"KE622x -- Set Output State.vi"("Resource In"=w354, "Check For SCPI Errors? (T)"=w351, "Output State"=w352, "error in (no error)"=w353) -> ("Resource Out (dupl)"=w349:refnum<visa-resource-name>, "error out"=w350:errorcluster)  [unwired: 10 in]
              }
              frame "On" {
                n75 = call <instrlib>:"KE622x -- Turn Output On And Check For Errors.vi"("Resource In"=w361, "Turn Off Output If Compliance?"="Turn Off Output If Voltage Limit?", "error in (no error)"=w360) -> ("Resource Out (dupl)"=w355:refnum<visa-resource-name>, "Interlock Tripped?"=w357:bool, "Compliance?"=w356:bool, "error out"=w358:errorcluster)  [unwired: 9 in]
              }
            }
            "Interlock Tripped?" <- w329
            "Voltage Limit?" <- w328
            n76 = Build Array(w312) -> (w311:T5[])
            n77 = TDMS Write(0:w308, 5:"6221" ("group name in (Untitled)"), 7:"Current Level" ("group name in (Untitled)"), 9:w311) -> (4:w309:refnum<k34>, 6:w310:string, 8:w294:string, 15:w306:errorcluster)  [unwired: 2 in]
            n78 = Get Date/Time In Seconds() -> (seconds since 1Jan1904=w300:timestamp)
            n79 = Build Array(w300) -> (w299:timestamp[])
            n80 = call <instrlib>:"KE622x -- Get Output State.vi"("Resource In"=w319, "error in (no error)"=w318) -> ("Resource Out (dupl)"=w316:refnum<visa-resource-name>, "Output State"=w304:T7, "error out"=w317:errorcluster)  [unwired: 11 in]
            n81 = Build Array(w304) -> (w303:T7[])
            n82 = TDMS Write(0:w309, 5:w310, 7:"Ouput State" ("group name in (Untitled)"), 9:w303, 11:w306) -> (4:w307:refnum<k34>, 6:w302:string, 15:w305:errorcluster)  [unwired: 1 in, 1 out]
            n83 = TDMS Write(0:w307, 5:w302, 7:"Time" ("group name in (Untitled)"), 9:w299, 11:w305) -> (4:w295:refnum<k34>, 6:w296:string, 15:w297:errorcluster)  [unwired: 1 in, 1 out]
            n84 = TDMS Set Properties(5:"Amps", 7:"Unit", 8:w297, 9:w294, 10:w296, 11:w295) -> (0:w290:errorcluster, 3:w291:refnum<k34>)  [unwired: 2 out]
            n85 = TDMS Flush(4:w290, 7:w291) -> ()  [unwired: 2 out]
            n86 = case shown="\"Off\", Default" w304 {
              tunnel: [FALSE TRUE] -> w315
              frame "Off", Default {
              }
              frame "On" {
              }
            }
            "Output on?" <- w315
            n87 = call <vilib>:"Simple Error Handler.vi"("error in (no error)"=w317) -> ("error out"=w320:errorcluster)  [unwired: 4 in, 4 out]
          }
          event "stop": Value Change {
            n88 = event-data() -> ("NewVal"=w362:bool)  [unwired: 1 in, 5 out]
          }
        }
      }
      n89 = Search and Replace String(input string=w140, search string=".vi") -> (result string=w143:string)  [unwired: 6 in, 3 out]
      n90 = property on="Tab Control" class="TabCtl (strict)"() -> ("Pages"=w139:refnum<vi>[])  [unwired: 2 in, 2 out]
      n91 = Index Array(array=w139, index=w135) -> (element=w138:refnum<vi>)
      n92 = call <instrlib>:"Configure Buffer.vi"("error in (no error)"=w146, "Buffer Source (0: None)"="Buffer Source (0: None)", "Buffer Size (2)"="Buffer Size (10)", "VISA resource name"=w147) -> ("error out"=w151:errorcluster, "VISA resource name out"=w150:refnum<visa-resource-name>)  [unwired: 6 in]
      n93 = property on="Property Node" class="Page"(reference=w138) -> ("PageLabel"=w137:string)  [unwired: 1 in, 2 out]
      n94 = Concatenate Strings(w143, " " ("string"), w137) -> (w130:string)
      n95 = call <instrlib>:"Configure Measurements.vi"("VISA resource name"=w150, "Measurement (0: Voltage Channel 1)"="Measurement (0: Voltage Channel 1) 2", "Integration Rate (5)"="Integration Rate (5)", "Integration Rate Units (0: Line Cycles)"="Integration Rate Units (0: Line Cycles)", "error in (no error)"=w151, "Sample Count (1)"="Buffer Size (10)") -> ("VISA resource name out"=w169:refnum<visa-resource-name>, "error out"=w170:errorcluster)  [unwired: 8 in]
      n96 = call "GenerateFilePaths.vi"("Device Name"=w130) -> ("Path"=w129:path)  [unwired: 4 in]
      n97 = TDMS Open(5:FALSE ("create index file? (T)"), 10:T21."open or create" ("operation (0:open)"), 11:w129) -> (0:w131:errorcluster, 3:w132:refnum<k34>)  [unwired: 4 in]
      "tdms file out" <- w132
      n98 = case shown="\"Voltage Settings\", Default" "Selected Measurement Settings" {
        tunnel: "Voltage Resolution (8) 2" -> [w210 _]
        tunnel: "Range Value (10) 2" -> [w211 _]
        tunnel: "Autorange (T: Enable) 2" -> [w212 _]
        tunnel: w170 -> [w216 w226]
        tunnel: w169 -> [w215 w225]
        tunnel: [w214 w224] -> w159
        tunnel: [w213 w223] -> w160
        tunnel: "Unit (0: Celsius)" -> [_ w222]
        tunnel: "Temperature Resolution (6)" -> [_ w221]
        tunnel: "Thermocouple Type (0: J)" -> [_ w220]
        tunnel: "Simulated Reference Temp (23 C)" -> [_ w219]
        tunnel: "Sensor (1: Internal)" -> [_ w218]
        tunnel: "Reference Junction Type (0: Internal)" -> [_ w217]
        tunnel: "Measurement (0: Voltage Channel 1) 2" -> [w209 _]
        frame "Voltage Settings", Default {
          n99 = call <instrlib>:"Configure Voltage Parameters.vi"("VISA resource name"=w215, "Measurement (1: Voltage Channel 1)"=w209, "Voltage Resolution (8)"=w210, "Range Value (12)"=w211, "Autorange (T: Enable)"=w212, "error in (no error)"=w216) -> ("VISA resource name out"=w214:refnum<visa-resource-name>, "error out"=w213:errorcluster)  [unwired: 8 in]
        }
        frame "Temp Settings" {
          n100 = call <instrlib>:"Configure Temperature Parameters.vi"("VISA resource name"=w225, "Sensor (0: Thermocouple)"=w218, "Reference Junction Type (0: Internal)"=w217, "Simulated Reference Temp (23 C)"=w219, "Thermocouple Type (0: J)"=w220, "Temperature Resolution (6)"=w221, "error in (no error)"=w226, "Unit (0: Celsius)"=w222) -> ("VISA resource name out"=w224:refnum<visa-resource-name>, "error out"=w223:errorcluster)  [unwired: 6 in]
        }
      }
      n101 = case shown="2" "Buffer Source (0: None)" {
        tunnel: w162 -> [_ w195]
        tunnel: "Math Calculation (0: Linear)" -> [_ w192]
        tunnel: w160 -> [w181 w194]
        tunnel: w159 -> [w180 w193]
        tunnel: "Use Input Signal as Target Value (F: Disable)" -> [_ w191]
        tunnel: "Target Value (1)" -> [_ w190]
        tunnel: "Offset Value (0)" -> [_ w187]
        tunnel: "Scale Factor (1)" -> [_ w186]
        tunnel: "Units (MX)" -> [_ w185]
        tunnel: [w181 w184] -> w133
        tunnel: [w180 w183] -> w134
        frame 0, Default {
        }
        frame 2 {
          n102 = call <instrlib>:"Configure Math Calculations.vi"("error in (no error)"=w194, "Math Calculation (0: Linear)"=w192, "Enable Math Calculation (F: Disable)"=w195, "VISA resource name"=w193) -> ("error out"=w189:errorcluster, "VISA resource name out"=w188:refnum<visa-resource-name>)  [unwired: 6 in]
          n103 = case shown="\"Percent Settings\"" "Selected Calculation Settings" {
            tunnel: w191 -> [_ w204]
            tunnel: w190 -> [_ w203]
            tunnel: w189 -> [w202 w205]
            tunnel: w188 -> [w201 w206]
            tunnel: w187 -> [w200 _]
            tunnel: w186 -> [w199 _]
            tunnel: w185 -> [w198 _]
            tunnel: [w197 w208] -> w184
            tunnel: [w196 w207] -> w183
            frame "Linear Settings", Default {
              n104 = call <instrlib>:"Configure Linear Math Calculation.vi"("Units (MX)"=w198, "error in (no error)"=w202, "Offset Value (0)"=w199, "Scale Factor (1)"=w200, "VISA resource name"=w201) -> ("error out"=w197:errorcluster, "VISA resource name out"=w196:refnum<visa-resource-name>)  [unwired: 5 in]
            }
            frame "Percent Settings" {
              n105 = call <instrlib>:"Configure Percent Math Calculation.vi"("error in (no error)"=w205, "Use Input Signal as Target Value (F: Disable)"=w204, "Target Value (1)"=w203, "VISA resource name"=w206) -> ("error out"=w208:errorcluster, "VISA resource name out"=w207:refnum<visa-resource-name>)  [unwired: 6 in]
            }
          }
        }
      }
      n106 = while {
        tunnel: w134 -> [w261]
        tunnel: w133 -> [w260]
        tunnel: w132 -> [w254]
        tunnel: w131 -> [w253]
        tunnel: [w235] -> w128
        tunnel: [w236] -> w127
        stop <- "stop" stop-if-true
        w231 = "Mean" ("group name in (Untitled)")
        w230 = "Raw" ("group name in (Untitled)")
        n107 = call <instrlib>:"Initiate.vi"("error in (no error)"=w260, "Initiate Type (0: Immediate)"="Initiate Type (0: Immediate)", "VISA resource name"=w261) -> ("error out"=w262:errorcluster, "VISA resource name out"=w263:refnum<visa-resource-name>)  [unwired: 7 in]
        n108 = call <instrlib>:"Read.vi"("error in (no error)"=w262, "VISA resource name"=w263) -> ("Measurements Metadata"=w229:T23, "Measurements"=w251:dbl[])  [unwired: 6 in, 2 out]
        "Measurements" <- w251
        n109 = TDMS Write(0:w254, 5:"2182a" ("group name in (Untitled)"), 7:w230, 9:w251, 11:w253) -> (4:w250:refnum<k34>, 6:w248:string, 15:w249:errorcluster)  [unwired: 1 in, 1 out]
        n110 = Index Array(array=w229) -> (element=→"Measurement Metadata":T6)  [unwired: 1 in]
        n111 = Build Array(w247) -> (w246:dbl[])
        n112 = TDMS Write(0:w250, 5:w248, 7:w231, 9:w246, 11:w249) -> (4:w245:refnum<k34>, 6:w243:string, 15:w244:errorcluster)  [unwired: 1 in, 1 out]
        n113 = Build Array(w242) -> (w241:timestamp[])
        n114 = property on="Measurement Metadata" class="Clust (strict)"() -> ("Controls[]"=w227:refnum<vi>[])  [unwired: 2 in, 2 out]
        n115 = TDMS Write(0:w245, 5:w243, 7:"Time" ("group name in (Untitled)"), 9:w241, 11:w244) -> (4:w239:refnum<k34>, 6:w232:string, 15:w238:errorcluster)  [unwired: 1 in, 1 out]
        n116 = flat-sequence {
          tunnel: w251 -> [w280]
          tunnel: [w279] -> w257
          tunnel: [w278] -> w256
          tunnel: [w279] -> w247
          tunnel: [w278] -> w242
          frame #0 {
            n117 = call-poly <vilib>:"Mean.vi"("X"=w280) -> ("mean"=w279:dbl)  [unwired: 1 out]
            n118 = Get Date/Time In Seconds() -> (seconds since 1Jan1904=w278:timestamp)
          }
        }
        n119 = TDMS Flush(4:w238, 7:w239) -> (0:w234:errorcluster, 3:w233:refnum<k34>)
        n120 = for {
          tunnel: w232 -> [w271]
          tunnel: w231 -> [w270]
          tunnel: w230 -> [w269]
          shift-right: [w277] -> w236
          shift-left: w234 -> [w273]
          shift-right: [w276] -> w235
          shift-left: w233 -> [w272]
          tunnel: w227 -> [w267] mode=indexing
          n121 = property class="Ctl"(reference=w267) -> ("Label.Text"=w266:string)  [unwired: 1 in, 2 out]
          n122 = property class="Ctl"(reference=w267) -> ("Value"=w265:variant)  [unwired: 1 in, 2 out]
          n123 = TDMS Set Properties(5:w265, 7:w266, 8:w273, 9:w270, 10:w271, 11:w272) -> (0:w274:errorcluster, 2:w268:string, 3:w275:refnum<k34>)  [unwired: 1 out]
          n124 = TDMS Set Properties(5:w265, 7:w266, 8:w274, 9:w269, 10:w268, 11:w275) -> (0:w277:errorcluster, 3:w276:refnum<k34>)  [unwired: 2 out]
        }
        n125 = To Double Precision Float(number=w256) -> (double precision float=w255:dbl)
        n126 = call "Build XY Graph2"("Reset"=FALSE, "Y Input"=w257, "X Input"=w255) -> ("XY Graph"=→"XY Graph 2":cluster{"X":dbl[], "Y":dbl[]}[])  [unwired: 7 in, 1 out]
      }
      n127 = call <instrlib>:"Close.vi"("VISA resource name"=w176, "error in (no error)"=w177) -> ()  [unwired: 13 in, 1 out]
      n128 = TDMS Close(8:w127, 11:w128) -> ()  [unwired: 2 out]
    }
  }
